vi "Acquire.vi"(8 "error in (no error)":errorcluster, 9 "Data Queue":refnum<queue>, 10 "Data Notifier":refnum<notifier>, 11 "Hardware Resources in":T1) -> (0 "error out":errorcluster, 3 "Hardware Resources out":T1)   [LabVIEW 2018, in "Acquisition.lvlib"]
doc: "Perform the acquisition. Replace the contents of this diagram with calls to acquisition hardware."
uses:
  Acquisition.lvlib
  Hardware Configuration.ctl
  Signal Type.ctl
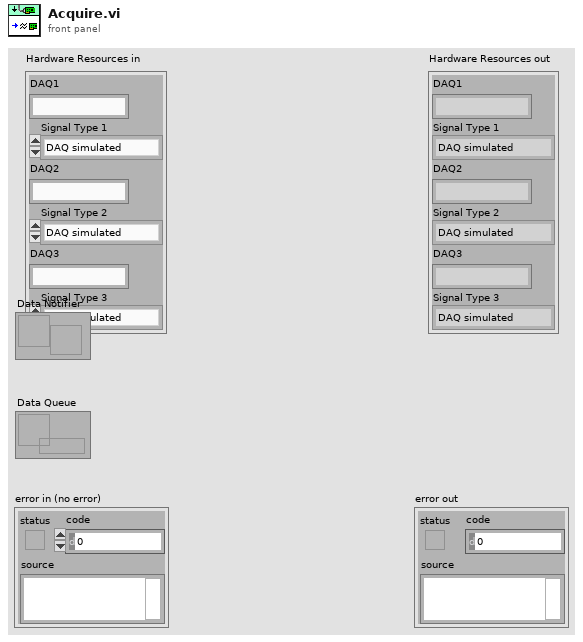
[diagram p1: front panel]
types:
  T1 = typedef "Acquisition.lvlib/Hardware Configuration.ctl" = cluster{"DAQ1":string, "Signal Type 1":T2, "DAQ2":string, "Signal Type 2":T2, "DAQ3":string, "Signal Type 3":T2}
  T2 = typedef "Acquisition.lvlib/Signal Type.ctl" = enum16{"DAQ simulated", "Sine and square wave", "Sine wave"}
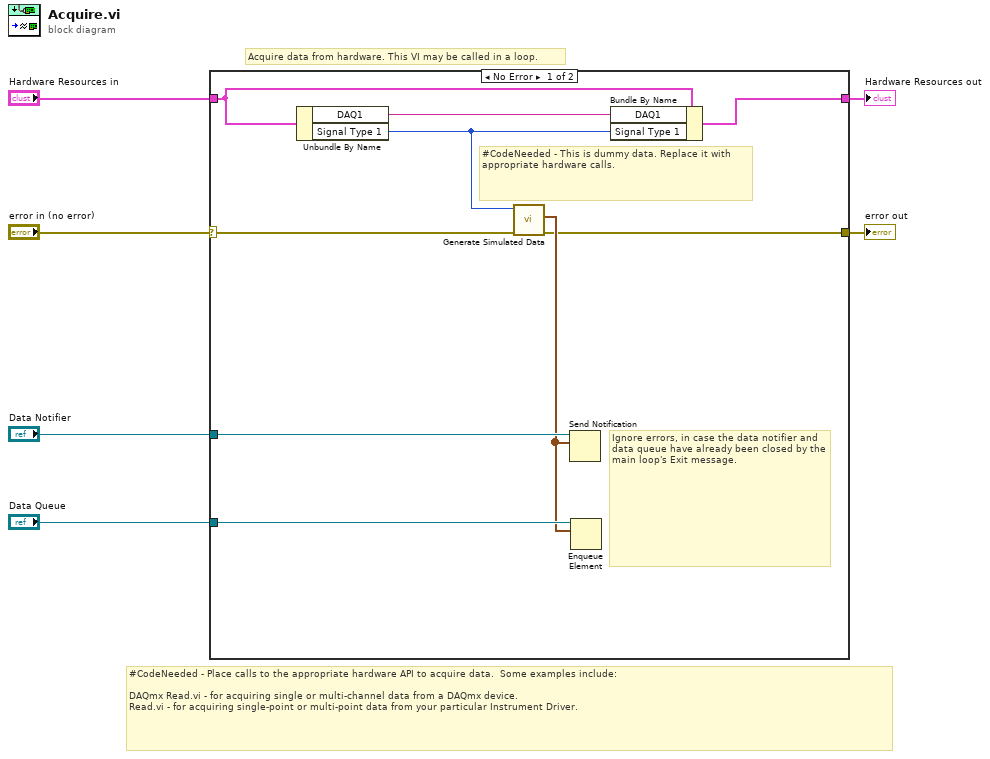
[diagram p0: block diagram]
diagram:
  # "Acquire data from hardware. This VI may be called in a loop."
  # "#CodeNeeded - Place calls to the appropriate hardware API to acquire data.  Some examples include:\n\nDAQmx Read.vi - for acquiring single or multi-channel data from a DAQmx device.\nRead.vi - for acquiring single-point or multi-point data from your particular Instrument Driver."
  n1 = case shown="No Error" "error in (no error)" {
    selector: "error in (no error)" -> [w14 w16]
    tunnel: [w7 w16] -> w5
    tunnel: "Hardware Resources in" -> [w11 w17]
    tunnel: [w15 w17] -> w3
    tunnel: "Data Notifier" -> [w10 _]
    tunnel: "Data Queue" -> [w9 _]
    frame No Error {
      # "Ignore errors, in case the data notifier and data queue have already been closed by the main loop's Exit message."
      # "#CodeNeeded - This is dummy data. Replace it with appropriate hardware calls."
      n2 = Unbundle By Name(w11) -> ("DAQ1"=w12:string, "Signal Type 1"=w13:T2)
      n3 = call "Generate Simulated Data.vi"("error in (no error)"=w14, "Signal Type"=w13) -> ("error out"=w7:errorcluster, "Graph Data"=w8:waveform(dbl)[])  [unwired: 8 in]
      n4 = Send Notification(notification=w8, notifier=w10) -> ()  [unwired: 1 in, 2 out]
      n5 = Enqueue Element(queue=w9, element=w8) -> ()  [unwired: 2 in, 3 out]
      n6 = Bundle By Name(cluster=w11, "DAQ1"=w12, "Signal Type 1"=w13) -> (w15:T1)
    }
    frame Error {
    }
  }
  "Hardware Resources out" <- w3
  "error out" <- w5
